vi "Add Label with Parameters.vi"(8 "error in":errorcluster, 10 "label":T2, 11 "port ref":T1 format="%.0x") -> (0 "error out":errorcluster, 3 "port ref out":T1 format="%.0x")   [LabVIEW 2020, in "Ballard ARINC 429 Scripting.lvlib"]
uses:
  Ballard ARINC 429 Scripting.lvlib
  <vilib>/NI VeriStand/Custom Device API/Custom Device Item Ref.ctl
  Shared/VS Channels Definition for Label.ctl
  Shared/VS Channel Definition for Parameter.ctl
  Shared/Direction.ctl
  Shared/Parameter Definition.ctl
  Encoding and Decoding/Encoding.ctl
  Shared/Transfer Type.ctl
  Shared/SDI.ctl
  <vilib>/NI VeriStand/Custom Device API/Custom Device API.lvlib
  Encoding and Decoding/Encoding and Decoding.lvlib
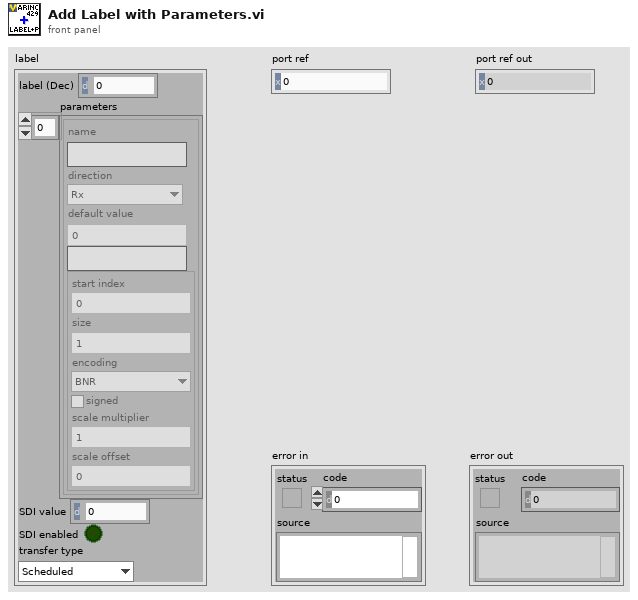
[diagram p1: front panel]
types:
  T1 = typedef "Custom Device API.lvlib/Custom Device Item Ref.ctl" = u64
  T2 = typedef "VS Channels Definition for Label.ctl" = cluster{"label (Dec)":u32, "parameters":T3[], "SDI value":u8, "SDI enabled":bool, "transfer type":T7}
  T3 = typedef "VS Channel Definition for Parameter.ctl" = cluster{"name":string, "direction":T4, "default value":dbl, "unit":string, "Parameter":T5}
  T4 = typedef "Direction.ctl" = enum16{"Rx", "Tx"}
  T5 = typedef "Parameter Definition.ctl" = cluster{"start index":i32, "size":i32, "encoding":T6, "signed":bool, "scale multiplier":dbl, "scale offset":dbl}
  T6 = typedef "Encoding and Decoding.lvlib/Encoding.ctl" = enum16{"BNR", "BCD", "Discrete"}
  T7 = typedef "Transfer Type.ctl" = enum16{"Scheduled", "Acyclic", "Block", "Strobe"}
  T8 = typedef "SDI.ctl" = i32
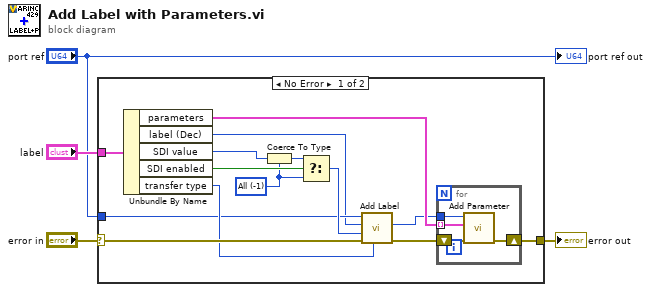
[diagram p0: block diagram]
diagram:
  n1 = case shown="No Error" "error in" {
    selector: "error in" -> [w18 w23]
    tunnel: "port ref" -> [w7 _]
    tunnel: [w17 w23] -> w4
    tunnel: "label" -> [w16 _]
    frame No Error {
      w10 = T8 -1 items=["All"=-1, "0 (b00)"=0, "1 (b01)"=1, "2 (b10)"=2, "3 (b11)"=3] ("SDI value")
      n2 = Unbundle By Name(w16) -> ("parameters"=w14:T3[], "label (Dec)"=w6:u32, "SDI value"=w12:u8, "SDI enabled"=w13:bool, "transfer type"=w8:T7)
      n3 = Coerce To Type(0:w12, 1:w10) -> (2:w11:T8)
      n4 = Select(t=w11, s=w13, f=w10) -> (s? t:f=w9:T8)
      n5 = call "Add Label.vi"("transfer type"=w8, "error in"=w18, "SDI value"=w9, "label (dec)"=w6, "port ref"=w7) -> ("error out"=w15:errorcluster, "label ref"=w5:T1)  [unwired: 4 in, 1 out]
      n6 = for {
        shift-right: [w20] -> w17
        shift-left: w15 -> [w21]
        tunnel: w14 -> [w19] mode=indexing
        tunnel: w5 -> [w22]
        n7 = call "Add Parameter.vi"("error in"=w21, "parameter"=w19, "label ref"=w22) -> ("error out"=w20:errorcluster)  [unwired: 6 in, 2 out]
      }
    }
    frame Error {
    }
  }
  "error out" <- w4
  "port ref out" <- "port ref"
